vi "Setup UI.vi"(8 "error in":errorcluster, 10 "Set UI to input? (F)":bool, 11 "Magnetic Field.lvclass":refnum<class "Magnetic Field.lvclass">) -> (0 "error out":errorcluster, 3 "Magnetic Field.lvclass out":refnum<class "Magnetic Field.lvclass">)   [LabVIEW 2015, in "Magnetic Field.lvclass"]
uses:
  Magnetic Field.lvclass
  Magnetic Field.lvclass/Magnetic Field.ctl
panel:
  in  "Sweep Rate":dbl[unit]
  # "Sweep Rate won't do anything\nuntil \"Scan Setup.vi\" is implemented\nfor this class"
  # "1"
  # "2"
  # "Magnetic Field Scan"
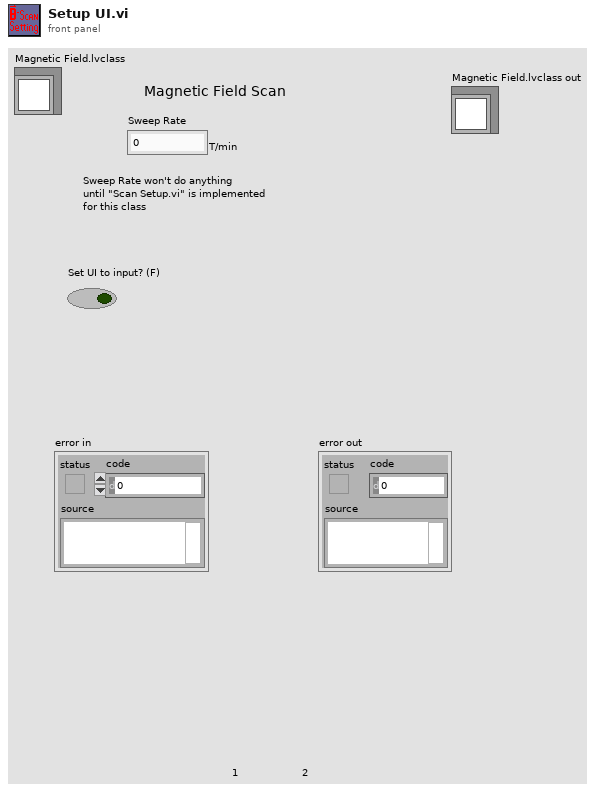
[diagram p1: front panel]
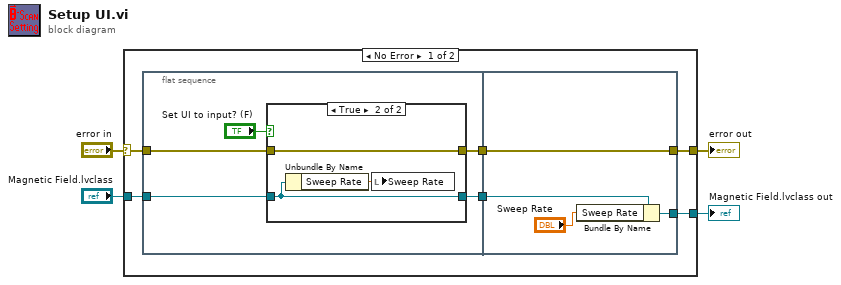
[diagram p0: block diagram]
diagram:
  n1 = case shown="No Error" "error in" {
    selector: "error in" -> [w8 w25]
    tunnel: [w10 w25] -> w3
    tunnel: [w7 w26] -> w2
    tunnel: "Magnetic Field.lvclass" -> [w5 w26]
    frame No Error {
      n2 = flat-sequence {
        tunnel: [w14] -> w9
        tunnel: w8 -> [w13]
        tunnel: [w12] -> w6
        tunnel: w5 -> [w11]
        tunnel: [w21] -> w10
        tunnel: w9 -> [w21]
        tunnel: [w23] -> w7
        tunnel: w6 -> [w24]
        frame #0 {
          n3 = case shown="True" "Set UI to input? (F)" {
            tunnel: [w17 w18] -> w14
            tunnel: w13 -> [w17 w18]
            tunnel: [w16 w20] -> w12
            tunnel: w11 -> [w16 w20]
            frame False {
            }
            frame True {
              n4 = Unbundle By Name(w20) -> ("Sweep Rate"=w19:dbl[unit])
              n5 = local write "Sweep Rate"(w19) -> ()
            }
          }
        }
        frame #1 {
          n6 = Bundle By Name(cluster=w24, "Sweep Rate"="Sweep Rate") -> (w23:refnum<class "Magnetic Field.lvclass">)
        }
      }
    }
    frame Error {
    }
  }
  "Magnetic Field.lvclass out" <- w2
  "error out" <- w3
